vi "ProdaNG.Tree.TestValues.Add.vi"(4 "TS":T1, 5 "TS":i32, 6 "Mode":T4, 7 "TestStepsTree":refnum<vi>, 8 "error in (no error)":errorcluster, 9 "units":T3[](array[typedef]), 10 "testStepId":i32, 11 "dbHandleIn":i32) -> (0 "error out":errorcluster, 1 "#changes":i32, 2 "TestStepValues":T5[](array[typedef]) {"minimum" format="%#.3f"; "maximum" format="%#.3f"}, 3 "dbHandle":i32)   [LabVIEW 2016]
doc: "This function returns a product structure for a product, which is identified by a part and a serial number.\nImportant information: The field 'individual' was taken over from the field 'allgemein' of the legacy data directly. Because of this most products have the value 0 further on and only a few the value 1. \nParameter:\nhandle is an Integer, which is returned by the function Login() at the creation of a new connection.\nwabcoPartId is the Id of the part.\nserialNumber is the serial number of the product for the part above.\nproduct is a pointer on a product structure, which is filled if the returncode is 0. The structure must be defined in the calling program.\n\nReturncodes:\n0 No error\n< 0 ORACLE Error code\n6 (ERROR_INVALID_HANDLE) in case of an invalid handle\n1403 Record does not exist"
uses:
  Controls/ProdaNG.TestValue.ctl
  ProdaNG.Tree.TestViewMode.ctl
  Controls/ProdaNG.UnitSimple.ctl
  ProdaNG.File.Step.ctl
  ProdaNG.Tree.Fglb.Value.ctl
  ProdaNG.Tree.Fglb.Data.ctl
  ProdaNG.Tree.Fglb.Element.ctl
  ProdaNG.Tree.Fglb.Action.ctl
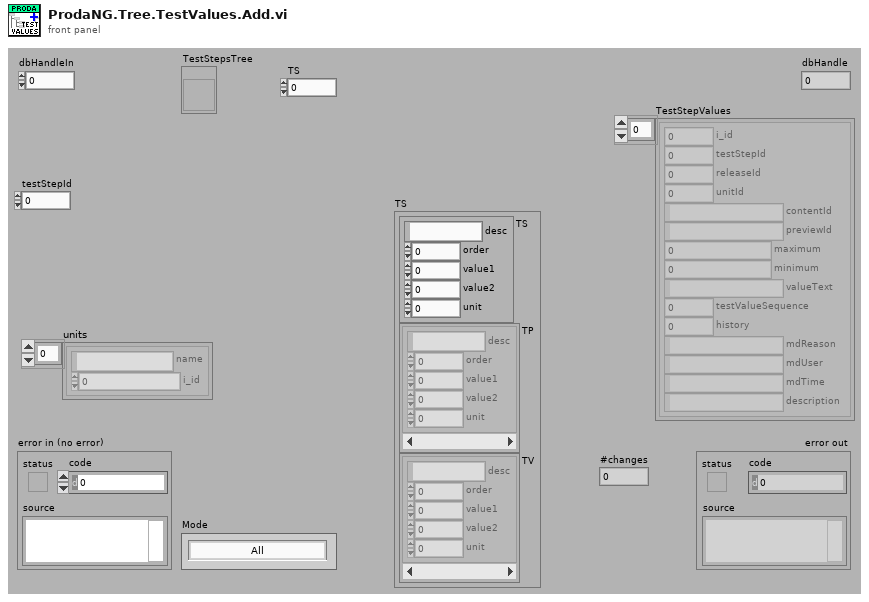
[diagram p1: front panel]
types:
  T1 = typedef "ProdaNG.File.Step.ctl" = cluster{"TS":T2, "TP":T2[], "TV":T2[]}
  T2 = typedef "ProdaNG.Tree.Fglb.Value.ctl" = cluster{"desc":string, "order":i32, "value1":dbl, "value2":dbl, "unit":i32}
  T3 = typedef "ProdaNG.UnitSimple.ctl" = cluster{"name":string, "i_id":i32}
  T4 = typedef "ProdaNG.Tree.TestViewMode.ctl" = enum16{"All", "Released", "Unreleased"}
  T5 = typedef "ProdaNG.TestValue.ctl" = cluster{"i_id":i32, "testStepId":i32, "releaseId":i32, "unitId":i32, "contentId":string, "previewId":string, "maximum":dbl, "minimum":dbl, "valueText":string, "testValueSequence":i32, "history":i32, "mdReason":string, "mdUser":string, "mdTime":string, "description":string}
  T6 = typedef "ProdaNG.Tree.Fglb.Action.ctl" = enum16{"init", "add", "get by row", "get by tag", "get by idx"}
  T7 = typedef "ProdaNG.Tree.Fglb.Element.ctl" = enum16{"-", "PP", "TS", "TP", "TV"}
  T8 = typedef "ProdaNG.Tree.Fglb.Data.ctl" = cluster{"tag":string, "row":i32, "element":T7, "idx1":i32, "idx2":i32, "file":bool}
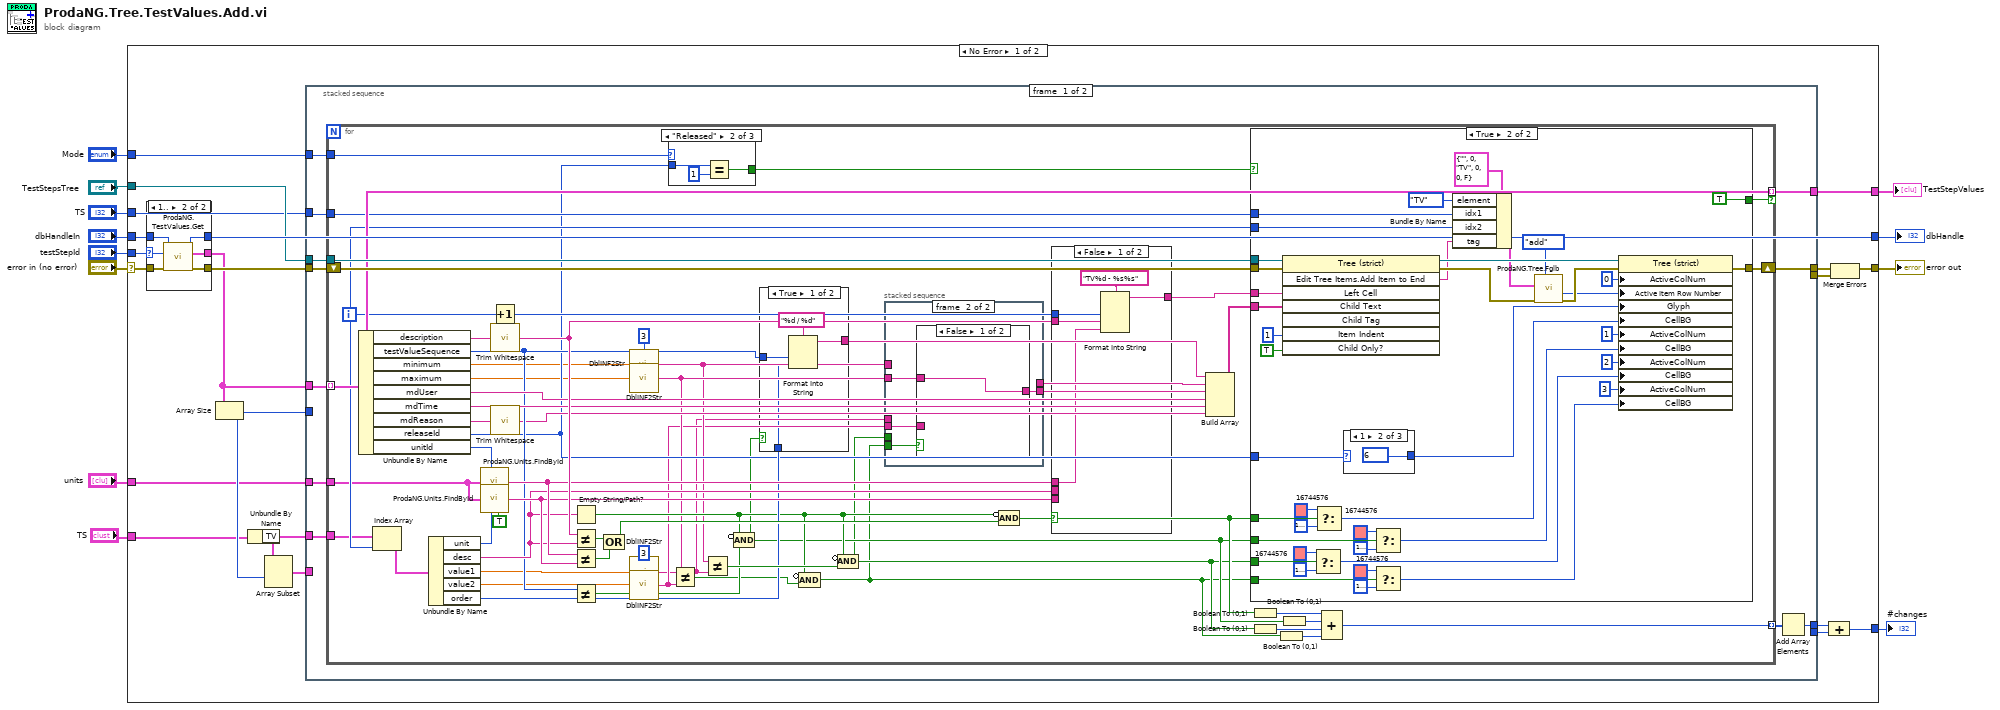
[diagram p0: block diagram]
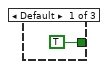
[diagram p3: hidden frame]
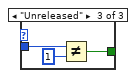
[diagram p4: hidden frame]
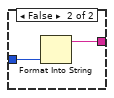
[diagram p5: hidden frame]
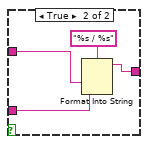
[diagram p7: hidden frame]
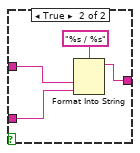
[diagram p8: hidden frame]
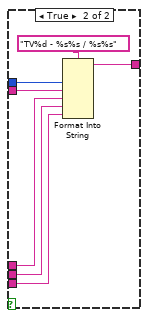
[diagram p9: hidden frame]
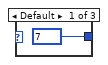
[diagram p11: hidden frame]
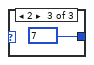
[diagram p12: hidden frame]
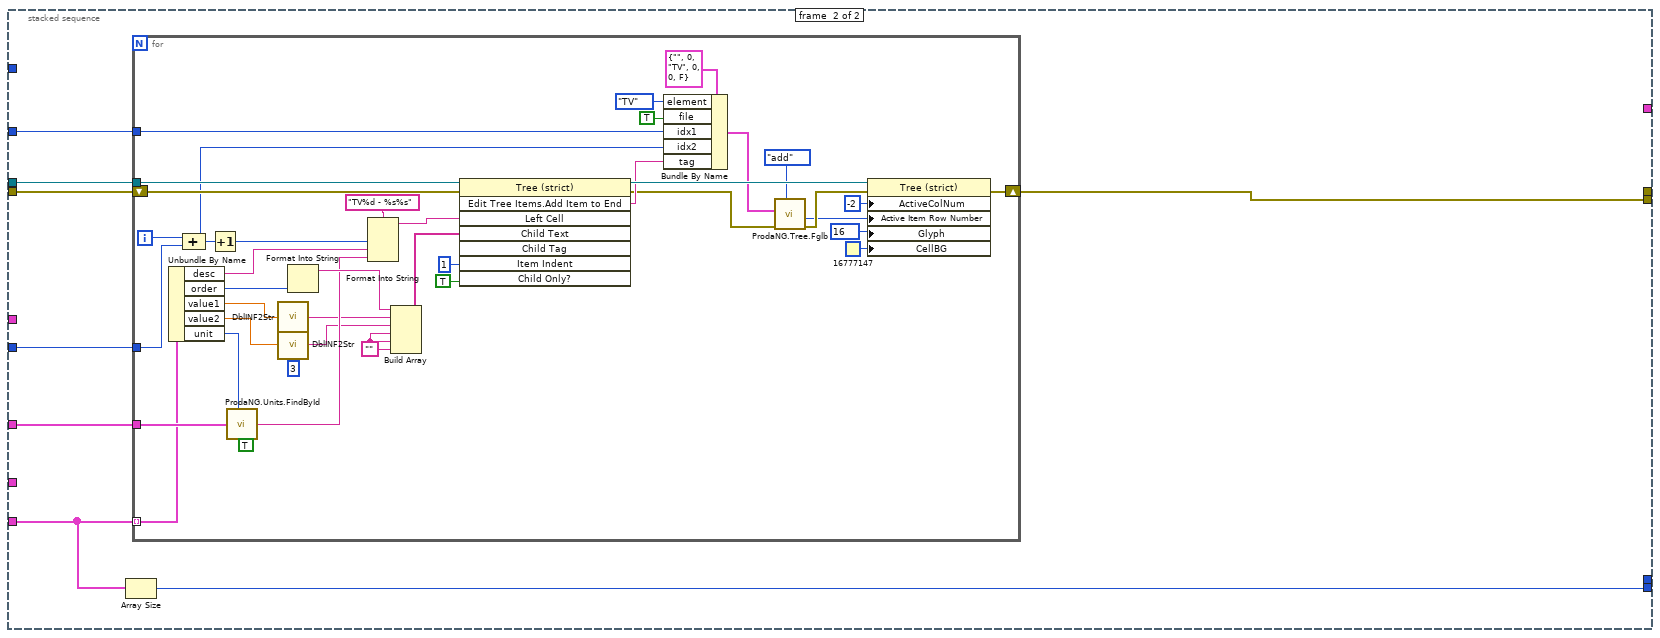
[diagram p13: hidden frame]
diagram:
  n1 = case shown="No Error" "error in (no error)" {
    selector: "error in (no error)" -> [w33 w249]
    tunnel: [w20 w249] -> w9
    tunnel: "dbHandleIn" -> [w32 w248]
    tunnel: [w31 w248] -> w8
    tunnel: "testStepId" -> [w16 _]
    tunnel: "TestStepsTree" -> [w28 _]
    tunnel: "TS" -> [w27 _]
    tunnel: "Mode" -> [w26 _]
    tunnel: [w19 _] -> w4
    tunnel: "units" -> [w23 _]
    tunnel: "TS" -> [w18 _]
    tunnel: [w13 _] -> w1
    frame No Error {
      n2 = case shown="1.." w16 {
        selector: w16 -> [_ w36]
        tunnel: w33 -> [w34 w41]
        tunnel: w32 -> [w35 w40]
        tunnel: [w35 w39] -> w31
        tunnel: [w34 w38] -> w29
        tunnel: [_ w37] -> w17
        frame Default {
        }
        frame 1.. {
          n3 = call "ProdaNG.TestValues.Get.vi"("error in (no error)"=w41, "testStepId"=w36, "dbHandleIn"=w40) -> ("error out"=w38:errorcluster, "TestStepValues"=w37:T5[], "dbHandle"=w39:i32)  [unwired: 6 in]
        }
      }
      n4 = Array Size(array=w17) -> (size(s)=w25:i32)
      n5 = Unbundle By Name(w18) -> ("TV"=w30:T2[])
      n6 = Array Subset(array=w30, index=w25) -> (w24:T2[])  [unwired: 1 in]
      n7 = stacked-sequence {
        tunnel: [w52 _] -> w22
        tunnel: w29 -> [w51 w207]
        tunnel: w28 -> [w50 w206]
        tunnel: w26 -> [w49 _]
        tunnel: [w48 _] -> w19
        tunnel: w23 -> [w47 w205]
        tunnel: w30 -> [w46 _]
        tunnel: w17 -> [w45 _]
        tunnel: w24 -> [_ w202]
        tunnel: w25 -> [_ w201]
        tunnel: w27 -> [w44 w204]
        tunnel: [_ w203] -> w21
        tunnel: [w42 _] -> w15
        tunnel: [_ w200] -> w14
        frame #0 {
          n8 = for {
            shift-right: [w106] -> w52
            shift-left: w51 -> [w111]
            tunnel: w45 -> [w103] mode=indexing
            tunnel: w50 -> [w109]
            tunnel: w49 -> [w76]
            tunnel: [w103] -> w48 mode=indexing if=w102
            tunnel: w47 -> [w93]
            tunnel: w46 -> [w99]
            tunnel: w44 -> [w85]
            tunnel: [w54] -> w43 mode=indexing
            i -> [w100]
            w53 = TRUE ("add quotas (F)")
            w65 = i16 3 ("precision (6)")
            w68 = i16 3 ("precision (6)")
            n9 = Unbundle By Name(w103) -> ("description"=w101:string, "testValueSequence"=w82:i32, "minimum"=w71:dbl, "maximum"=w72:dbl, "mdUser"=w83:string, "mdTime"=w84:string, "mdReason"=w108:string, "releaseId"=w77:i32, "unitId"=w95:i32)
            n10 = Index Array(array=w99, index=w100) -> (element=w73:T2)
            n11 = Unbundle By Name(w73) -> ("unit"=w94:i32, "desc"=w89:string, "value1"=w66:dbl, "value2"=w67:dbl, "order"=w86:i32)
            n12 = call "ProdaNG.Units.FindById.vi"("units"=w93, "unit id"=w95, "add brackets (F)"=w53) -> ("unit str"=w92:string)
            n13 = call "ProdaNG.Units.FindById.vi"("units"=w93, "unit id"=w94, "add brackets (F)"=w53) -> ("unit str"=w91:string)
            n14 = Increment(x=w100) -> (x+1=w107:i32)
            n15 = call <vilib>:"Trim Whitespace.vi"("string"=w101) -> ("trimmed string"=w98:string)  [unwired: 1 in]
            n16 = call <vilib>:"Trim Whitespace.vi"("string"=w108) -> ("trimmed string"=w78:string)  [unwired: 1 in]
            n17 = Empty String/Path?(string/path=w89) -> (empty?=w80:bool)
            n18 = Not Equal?(x=w98, y=w89) -> (x != y?=w97:bool)
            n19 = Not Equal?(x=w92, y=w91) -> (x != y?=w96:bool)
            n20 = Not Equal?(x=w82, y=w86) -> (x != y?=w87:bool)
            n21 = Compound Arithmetic op=OR(w97, w96) -> (w90:bool)
            n22 = call "DblINF2Str.vi"("Numeric"=w71, "precision (6)"=w68) -> ("string"=w69:string)
            n23 = call "DblINF2Str.vi"("Numeric"=w72, "precision (6)"=w68) -> ("string"=w70:string)
            n24 = call "DblINF2Str.vi"("Numeric"=w66, "precision (6)"=w65) -> ("string"=w63:string)
            n25 = call "DblINF2Str.vi"("Numeric"=w67, "precision (6)"=w65) -> ("string"=w64:string)
            n26 = case shown="\"Released\"" w76 {
              tunnel: w77 -> [_ w115 w118]
              tunnel: [TRUE w113 w116] -> w75
              frame Default {
              }
              frame "Released" {
                n27 = Equal?(x=w115, y=1) -> (x = y?=w113:bool)
              }
              frame "Unreleased" {
                n28 = Not Equal?(x=w118, y=1) -> (x != y?=w116:bool)
              }
            }
            n29 = Not Equal?(x=w70, y=w64) -> (x != y?=w81:bool)
            n30 = Not Equal?(x=w69, y=w63) -> (x != y?=w88:bool)
            n31 = Compound Arithmetic op=AND(invert w80, w87) -> (w60:bool)
            n32 = case shown="True" w60 {
              tunnel: w82 -> [w122 w124]
              tunnel: [w121 w123] -> w105
              tunnel: w86 -> [w119 _]
              frame True {
                n33 = Format Into String(format string="%d / %d", w122, w119) -> (resulting string=w121:string)  [unwired: 2 in, 1 out]
              }
              frame False {
                n34 = Format Into String(w124) -> (resulting string=w123:string)  [unwired: 3 in, 1 out]
              }
            }
            n35 = Compound Arithmetic op=AND(invert w80, w81) -> (w57:bool)
            n36 = Compound Arithmetic op=AND(invert w80, w88) -> (w58:bool)
            n37 = stacked-sequence {
              tunnel: w63 -> [w128 _]
              tunnel: w58 -> [w127 _]
              tunnel: w69 -> [w126 _]
              tunnel: [w125 _] -> w79
              tunnel: w70 -> [_ w137]
              tunnel: w64 -> [_ w136]
              tunnel: [_ w135] -> w74
              tunnel: w57 -> [_ w134]
              frame #0 {
                n38 = case shown="False" w127 {
                  tunnel: [w129 w132] -> w125
                  tunnel: w126 -> [w129 w131]
                  tunnel: w128 -> [_ w130]
                  frame False {
                  }
                  frame True {
                    n39 = Format Into String(format string="%s / %s", w131, w130) -> (resulting string=w132:string)  [unwired: 2 in, 1 out]
                  }
                }
              }
              frame #1 {
                n40 = case shown="False" w134 {
                  tunnel: [w138 w141] -> w135
                  tunnel: w137 -> [w138 w140]
                  tunnel: w136 -> [_ w139]
                  frame False {
                  }
                  frame True {
                    n41 = Format Into String(format string="%s / %s", w140, w139) -> (resulting string=w141:string)  [unwired: 2 in, 1 out]
                  }
                }
              }
            }
            n42 = Compound Arithmetic op=AND(invert w80, w90) -> (w62:bool)
            n43 = case shown="False" w62 {
              tunnel: w92 -> [w143 w150]
              tunnel: w107 -> [w146 w153]
              tunnel: w98 -> [w145 w152]
              tunnel: [w144 w151] -> w104
              tunnel: w89 -> [_ w149]
              tunnel: w91 -> [_ w148]
              frame False {
                n44 = Format Into String(format string="TV%d - %s%s", w146, w145, w143) -> (resulting string=w144:string)  [unwired: 2 in, 1 out]
              }
              frame True {
                n45 = Format Into String(format string="TV%d - %s%s / %s%s", w153, w152, w150, w149, w148) -> (resulting string=w151:string)  [unwired: 2 in, 1 out]
              }
            }
            n46 = Build Array(w105, w79, w74, w83, w84, w78) -> (w110:string[])
            n47 = case shown="True" w75 {
              tunnel: w111 -> [w155 w194]
              tunnel: w104 -> [_ w193]
              tunnel: w110 -> [_ w192]
              tunnel: w109 -> [_ w191]
              tunnel: [w155 w186] -> w106
              tunnel: w100 -> [_ w183]
              tunnel: [_ TRUE] -> w102
              tunnel: w62 -> [_ w177]
              tunnel: w60 -> [_ w171]
              tunnel: w58 -> [_ w166]
              tunnel: w85 -> [_ w163]
              tunnel: w77 -> [_ w162]
              tunnel: w57 -> [_ w159]
              frame False {
              }
              frame True {
                n48 = invoke on="Invoke Node" class="Tree (strict)" method="Edit Tree Items.Add Item to End"(reference=w191, error in=w194, "Left Cell"=w193, "Child Text"=w192, "Item Indent"=1 ("New Item Indentation"), "Child Only?"=TRUE) -> (reference out=w188:refnum<vi>, error out=w181:errorcluster, "Edit Tree Items:Add Item to End"=w178:string)  [unwired: 2 in, 5 out]
                n49 = Select(t=u32 16744576, s=w166, f=u32 16777225) -> (s? t:f=w165:u32)
                n50 = Select(t=u32 16744576, s=w177, f=u32 16777225) -> (s? t:f=w164:u32)
                n51 = case shown="1" w162 {
                  tunnel: [7 6 7] -> w156
                  frame Default {
                  }
                  frame 1 {
                  }
                  frame 2 {
                  }
                }
                n52 = Select(t=u32 16744576, s=w171, f=u32 16777225) -> (s? t:f=w170:u32)
                n53 = Select(t=u32 16744576, s=w159, f=u32 16777225) -> (s? t:f=w157:u32)
                n54 = Bundle By Name(cluster=T8 {"tag"="", "row"=0, "element"=enum."TV", "idx1"=0, "idx2"=0, "file"=FALSE} ("entry in"), "element"=ProdaNG.Tree.Fglb.Element."TV", "idx1"=w163, "idx2"=w183, "tag"=w178) -> (w182:T8)
                n55 = call "ProdaNG.Tree.Fglb.vi"("Action (add)"=ProdaNG.Tree.Fglb.Action."add", "error in"=w181, "entry in"=w182) -> ("error out"=w189:errorcluster, "active row"=w187:i32)  [unwired: 6 in, 1 out]
                n56 = property class="Tree (strict)"(reference=w188, error in=w189, "ActiveColNum"=0 ("Active Cell:Active Column Number"), "Active Item Row Number"=w187, "Glyph"=w156, "CellBG"=w164, "ActiveColNum"=1 ("Active Cell:Active Column Number"), "CellBG"=w170, "ActiveColNum"=2 ("Active Cell:Active Column Number"), "CellBG"=w165, "ActiveColNum"=3 ("Active Cell:Active Column Number"), "CellBG"=w157) -> (error out=w186:errorcluster)  [unwired: 1 out]
              }
            }
            n57 = Boolean To (0,1)(Boolean=w62) -> (0, 1=w61:i16)
            n58 = Boolean To (0,1)(Boolean=w58) -> (0, 1=w55:i16)
            n59 = Boolean To (0,1)(Boolean=w57) -> (0, 1=w56:i16)
            n60 = Boolean To (0,1)(Boolean=w60) -> (0, 1=w59:i16)
            n61 = Compound Arithmetic op=ADD(w61, w59, w55, w56) -> (w54:i16)
          }
          n62 = Add Array Elements(numeric array=w43) -> (sum=w42:i16)
        }
        frame #1 {
          n63 = Array Size(array=w202) -> (size(s)=w200:i32)
          n64 = for {
            shift-right: [w243] -> w203
            shift-left: w207 -> [w247]
            tunnel: w206 -> [w245]
            tunnel: w205 -> [w237]
            tunnel: w202 -> [w230] mode=indexing
            tunnel: w201 -> [w227]
            tunnel: w204 -> [w219]
            i -> [w239]
            w216 = i16 3 ("precision (6)")
            w217 = ""
            n65 = Unbundle By Name(w230) -> ("desc"=w240:string, "order"=w235:i32, "value1"=w213:dbl, "value2"=w210:dbl, "unit"=w238:i32)
            n66 = Compound Arithmetic op=ADD(w239, w227) -> (w209:i32)
            n67 = Increment(x=w209) -> (x+1=w244:i32)
            n68 = call "ProdaNG.Units.FindById.vi"("units"=w237, "unit id"=w238, "add brackets (F)"=TRUE ("add quotas (F)")) -> ("unit str"=w236:string)
            n69 = call "DblINF2Str.vi"("Numeric"=w213, "precision (6)"=w216) -> ("string"=w215:string)
            n70 = call "DblINF2Str.vi"("Numeric"=w210, "precision (6)"=w216) -> ("string"=w214:string)
            n71 = Format Into String(w235) -> (resulting string=w242:string)  [unwired: 3 in, 1 out]
            n72 = Format Into String(format string="TV%d - %s%s", w244, w240, w236) -> (resulting string=w241:string)  [unwired: 2 in, 1 out]
            n73 = Build Array(w242, w215, w214, w217, w217, w217) -> (w246:string[])
            n74 = invoke on="Invoke Node" class="Tree (strict)" method="Edit Tree Items.Add Item to End"(reference=w245, error in=w247, "Left Cell"=w241, "Child Text"=w246, "Item Indent"=1 ("New Item Indentation"), "Child Only?"=TRUE) -> (reference out=w231:refnum<vi>, error out=w211:errorcluster, "Edit Tree Items:Add Item to End"=w222:string)  [unwired: 2 in, 5 out]
            n75 = Bundle By Name(cluster=T8 {"tag"="", "row"=0, "element"=enum."TV", "idx1"=0, "idx2"=0, "file"=FALSE} ("entry in"), "element"=ProdaNG.Tree.Fglb.Element."TV", "file"=TRUE, "idx1"=w219, "idx2"=w209, "tag"=w222) -> (w212:T8)
            n76 = call "ProdaNG.Tree.Fglb.vi"("Action (add)"=ProdaNG.Tree.Fglb.Action."add", "error in"=w211, "entry in"=w212) -> ("error out"=w223:errorcluster, "active row"=w220:i32)  [unwired: 6 in, 1 out]
            n77 = property class="Tree (strict)"(reference=w231, error in=w223, "ActiveColNum"=-2 ("Active Cell:Active Column Number"), "Active Item Row Number"=w220, "Glyph"=16, "CellBG"=u32 16777147) -> (error out=w243:errorcluster)  [unwired: 1 out]
          }
        }
      }
      n78 = Compound Arithmetic op=ADD(w15, w14) -> (w13:i32)
      n79 = Merge Errors(w22, w21) -> (w20:errorcluster)
    }
    frame Error {
    }
  }
  "error out" <- w9
  "dbHandle" <- w8
  "TestStepValues" <- w4
  "#changes" <- w1
